vi "classify error.vi"(8 "error to classify":errorcluster, 11 "TDMS datalogger runtime in":refnum<class "TDMS datalogger runtime.lvclass">) -> (0 "classified error":errorcluster, 2 "error classification":T1, 3 "TDMS datalogger runtime out":refnum<class "TDMS datalogger runtime.lvclass">)   [LabVIEW 2013, in "TDMS datalogger runtime.lvclass"]
doc: "Allows a module to classify an error generated at any point during execution. This <b>error classification</b> can then be used by calling code to determine if execution can continue. In addition, this function can be used to allow a component to clear an error, convert an error to a warning, or attempt to recover from an error. Recovery may be attempted only if <b>attempt recovery?</b> is true."
uses:
  TDMS datalogger runtime.lvclass
  <vilib>/NI/Tag Bus Module Framework/runtime/error classification.ctl
  <vilib>/NI/Tag Bus Module Framework/runtime/TBM module execution interface.lvclass
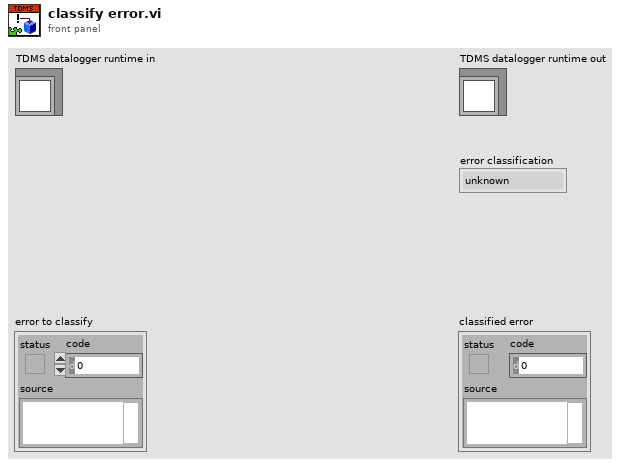
[diagram p1: front panel]
types:
  T1 = typedef "TBM module execution interface.lvclass/error classification.ctl" = enum16{"unknown", "none", "trivial", "recoverable", "critical"}
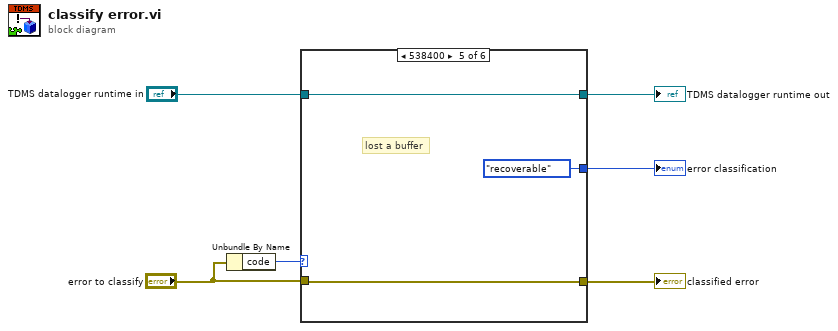
[diagram p0: block diagram]
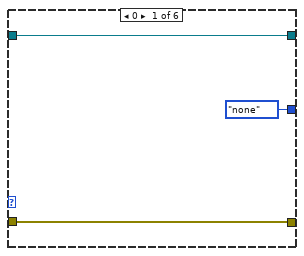
[diagram p2: hidden frame]
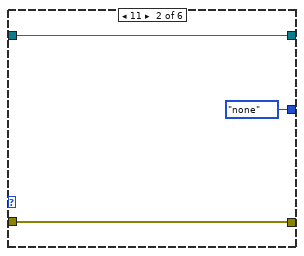
[diagram p3: hidden frame]
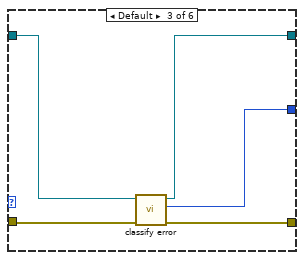
[diagram p4: hidden frame]
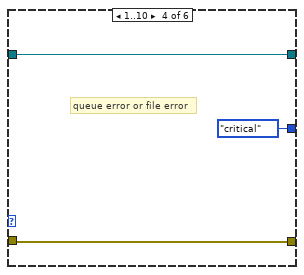
[diagram p5: hidden frame]
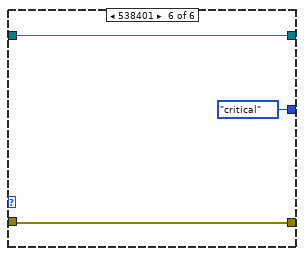
[diagram p6: hidden frame]
diagram:
  n1 = Unbundle By Name("error to classify") -> ("code"=w1:i32)
  n2 = case shown="538400" w1 {
    tunnel: "error to classify" -> [w8 w11 w17 w18 w21 w24]
    tunnel: [w8 w11 w16 w18 w21 w24] -> w3
    tunnel: [error_classification."none" ("error classification") error_classification."none" ("error classification") w15 error_classification."critical" ("error classification") error_classification."recoverable" ("error classification") error_classification."critical" ("error classification")] -> w2
    tunnel: "TDMS datalogger runtime in" -> [w9 w12 w14 w19 w22 w25]
    tunnel: [w9 w12 w13 w19 w22 w25] -> w5
    frame 0 {
    }
    frame 11 {
    }
    frame Default {
      n3 = call-parent "classify error.vi"("error to classify"=w17, "module in"=w14) -> ("classified error"=w16:errorcluster, "error classification"=w15:T1, "module out"=w13:refnum<class "TDMS datalogger runtime.lvclass">)  [unwired: 7 in]
    }
    frame 1..10 {
      # "queue error or file error"
    }
    frame 538400 {
      # "lost a buffer"
    }
    frame 538401 {
    }
  }
  "TDMS datalogger runtime out" <- w5
  "error classification" <- w2
  "classified error" <- w3
